vi "Delete.vi"(8 "에러 입력":errorcluster caption="에러 입력(에러 없음)") -> (0 "에러 출력":errorcluster)   [LabVIEW 2020]
uses:
  <vilib>/Utility/sysdir.llb/System Directory Type.ctl
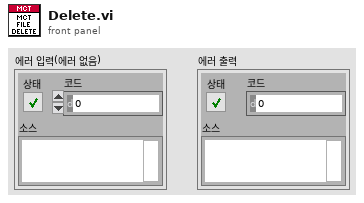
[diagram p1: front panel]
types:
  T1 = typedef "System Directory Type.ctl" = i32
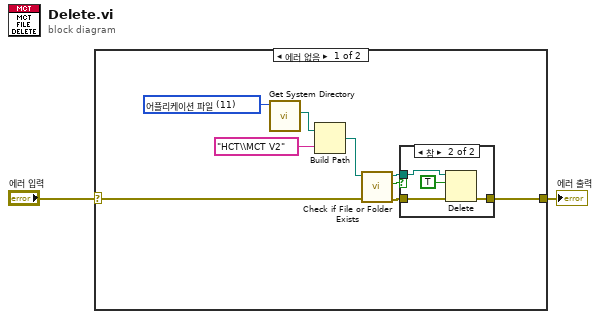
[diagram p0: block diagram]
diagram:
  n1 = case shown="에러 없음" "에러 입력" {
    selector: "에러 입력" -> [w4 w17]
    tunnel: [w3 w17] -> w2
    frame No Error {
      w11 = T1 11 items=["사용자 홈"=0, "사용자 데스크탑"=1, "사용자 문서"=2, "사용자 어플리케이션 데이터"=3, "사용자 환경"=4, "사용자 임시"=5, "퍼블릭 문서"=6, "퍼블릭 어플리케이션 데이터"=7, "퍼블릭 환경"=8, "퍼블릭 캐시"=13, "시스템 코어 라이브러리"=9, "시스템 설치된 라이브러리"=10, "어플리케이션 파일"=11, "부팅 볼륨 루트"=12] ("system directory type")
      n2 = call <vilib>:"Get System Directory.vi"("system directory type"=w11) -> ("system directory"=w10:path)  [unwired: 10 in]
      n3 = Build Path(base path=w10, name or relative path="HCT\\MCT V2" ("이름 또는 상대 경로")) -> (appended path=w8:path)
      n4 = call <vilib>:"Check if File or Folder Exists.vi"("error in (no error)"=w4, "path"=w8) -> ("error out"=w7:errorcluster, "file or folder exists?"=w5:bool, "dup path"=w6:path)  [unwired: 7 in]
      n5 = case shown="참" w5 {
        tunnel: [w12 w15] -> w3
        tunnel: w7 -> [w12 w14]
        tunnel: w6 -> [_ w13]
        frame False {
        }
        frame True {
          n6 = Delete(path (use dialog)=w13, entire hierarchy (F)=TRUE ("전체 계층구조(거짓)"), error in=w14) -> (error out=w15:errorcluster)  [unwired: 2 in, 2 out]
        }
      }
    }
    frame Error {
    }
  }
  "에러 출력" <- w2
